vi "Inches to Ticks.vi"(1 "Inches":dbl format="%#_13g") -> (0 "Ticks":dbl format="%#_13g")   [LabVIEW 2016]
panel:
  out "error out":errorcluster
  in  "error in":errorcluster
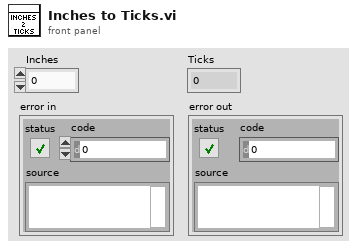
[diagram p1: front panel]
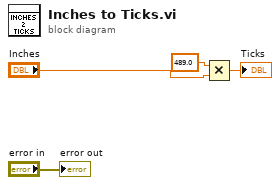
[diagram p0: block diagram]
diagram:
  n1 = Multiply(x=489.0, y="Inches") -> (x*y=→"Ticks":dbl)
  "error out" <- "error in"
